vi "APS Controller.vi"() -> ()   [LabVIEW 2025]
panel:
  in  "Polarity":enum16{"Positive", "Negative"}(ring)
  out "Current Setpoint":i32
  in  "APS PORT":refnum<visa-resource-name>="COM3"
  out "?":string
  out "error out":errorcluster
  out "Connected?":bool
  in  "Set current":i32
  in  "Set Voltage":i32
  in  "Measure Temp":bool
  in  "Measure AUX2":bool
  in  "Measure AUX1":bool
  in  "Connect":bool
  in  "Stop Button":bool
  in  "Measure Voltage":bool
  in  "Measure Current":bool
  in  "Set INT Mode":bool
  in  "Set Current":bool
  in  "Set PC Mode":bool
  in  "Set Voltage":bool
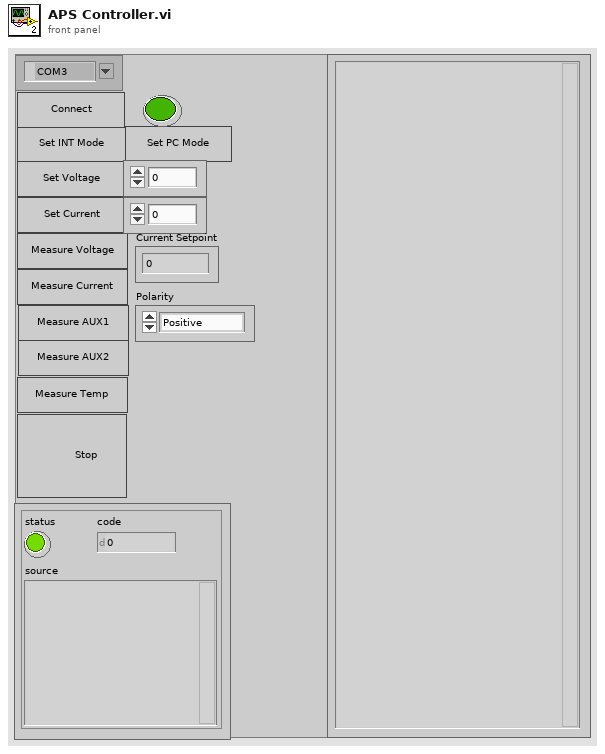
[diagram p1: front panel]
types:
  T1 = enum16{"1. Identify", "2. Control Mode", "3. Set PC Mode", "4. Set INT Mode", "5. Set Voltage", "6. Set Current", "7. Measure Voltage", "8. Measure Current", "9. Measure AUX1", "10. Measure AUX2", "11. Measure Temperature", "12. Switch Polarity"}
  T2 = cluster{"Task Type":enum16{"1. Identify", "2. Control Mode", "3. Set PC Mode", "4. Set INT Mode", "5. Set Voltage", "6. Set Current", "7. Measure Voltage", "8. Measure Current", "9. Measure AUX1", "10. Measure AUX2", "11. Measure Temperature", "12. Switch Polarity"}, "DBL Argument":i32, "BLN Argument":bool, "Task CMD":enum16{"*IDN?", "CONT MODE?", "CONT MODE PC", "CONT MODE INT", "SOUR VOLT ", "SOUR CURR ", "MEAS VOLT?", "MEAS CURR?", "MEAS AUX1?", "MEAS AUX2?", "MEAS TEMP?", "SOUR POLA"}, "CMD TYPE":enum16{"1. Timeout?", "2. New Current?", "3. User CMD"}, "Polarity":enum16{"POS ", "NEG "}}
  T3 = enum16{"*IDN?", "CONT MODE?", "CONT MODE PC", "CONT MODE INT", "SOUR VOLT ", "SOUR CURR ", "MEAS VOLT?", "MEAS CURR?", "MEAS AUX1?", "MEAS AUX2?", "MEAS TEMP?", "SOUR POLA"}
  T4 = enum16{"*IDN?", "CONT MODE?", "CONT MODE PC", "CONT MODE INT", "SOUR VOLT ", "SOUR CURR ", "MEAS VOLT?", "MEAS CURR?", "MEAS AUX1?", "MEAS AUX2?", "MEAS TEMP?"}
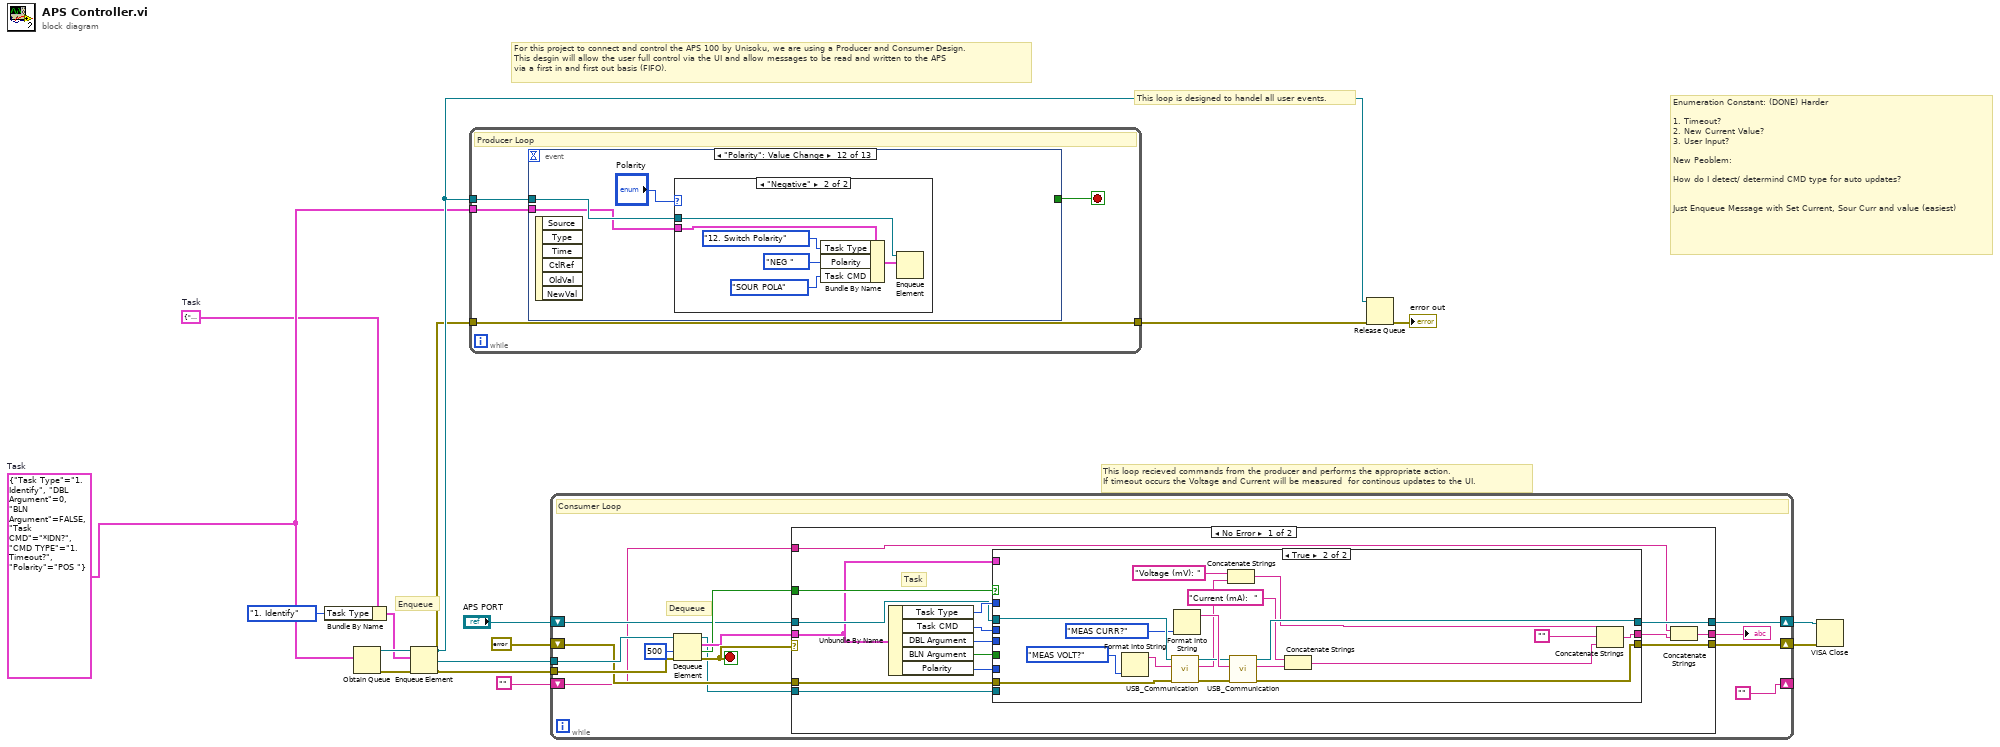
[diagram p0: block diagram]
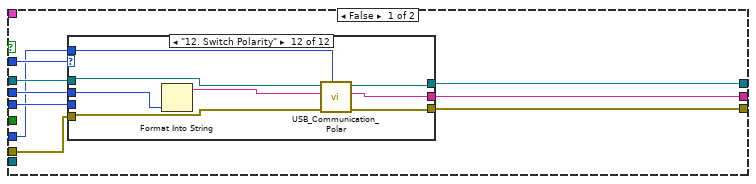
[diagram p2: hidden frame]
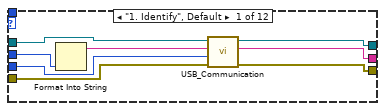
[diagram p3: hidden frame]
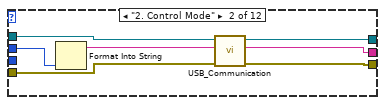
[diagram p4: hidden frame]
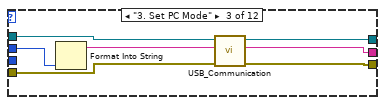
[diagram p5: hidden frame]
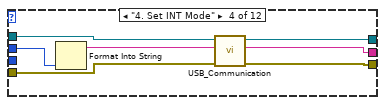
[diagram p6: hidden frame]
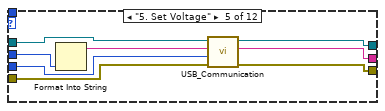
[diagram p7: hidden frame]
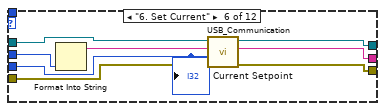
[diagram p8: hidden frame]
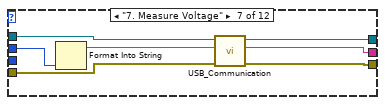
[diagram p9: hidden frame]
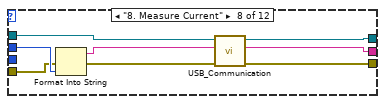
[diagram p10: hidden frame]
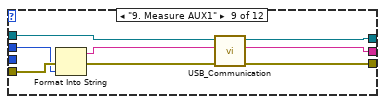
[diagram p11: hidden frame]
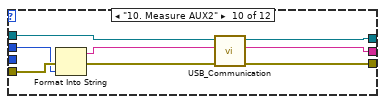
[diagram p12: hidden frame]
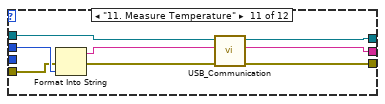
[diagram p13: hidden frame]
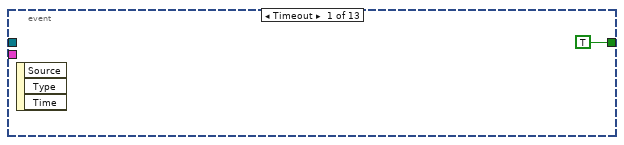
[diagram p15: hidden frame]
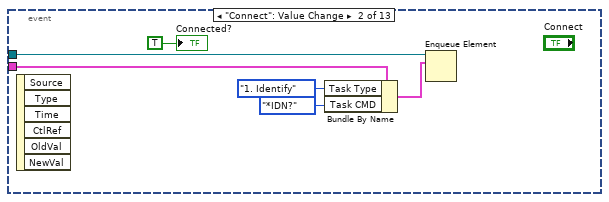
[diagram p16: hidden frame]
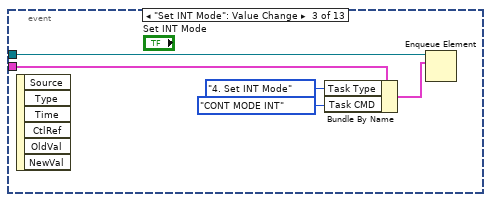
[diagram p17: hidden frame]
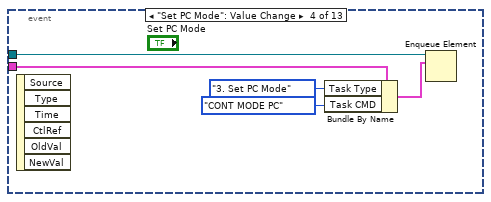
[diagram p18: hidden frame]
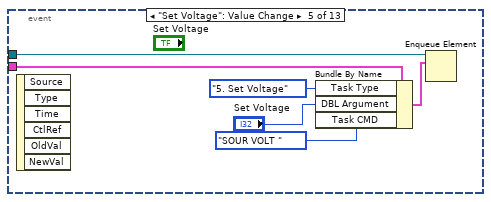
[diagram p19: hidden frame]
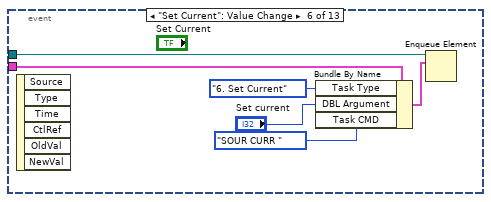
[diagram p20: hidden frame]
diagram:
  w3 = T2 {"Task Type"=enum."1. Identify", "DBL Argument"=0, "BLN Argument"=FALSE, "Task CMD"=enum."*IDN?", "CMD TYPE"=enum."1. Timeout?", "Polarity"=enum."POS "}  # Task
  w4 = T2 {"Task Type"=enum."1. Identify", "DBL Argument"=0, "BLN Argument"=FALSE, "Task CMD"=enum."*IDN?", "CMD TYPE"=enum."1. Timeout?", "Polarity"=enum."POS "}  # Task
  # "Enqueue"
  # "Enumeration Constant: (DONE) Harder\n\n1. Timeout?\n2. New Current Value?\n3. User Input? \n\nNew Peoblem:\n\nHow do I detect/ determind CMD type for auto updates?\n\n\nJust Enqueue Message with Set Current, Sour Curr and value (easiest)"
  # "This loop is designed to handel all user events."
  # "This loop recieved commands from the producer and performs the appropriate action.\nIf timeout occurs the Voltage and Current will be measured  for continous updates to the UI."
  # "For this project to connect and control the APS 100 by Unisoku, we are using a Producer and Consumer Design. \nThis desgin will allow the user full control via the UI and allow messages to be read and written to the APS\nvia a first in and first out basis (FIFO)."
  n1 = Bundle By Name(cluster=w3, "Task Type"=T1."1. Identify") -> (w1:T2)
  n2 = Obtain Queue(element data type=w4) -> (queue out=w5:refnum<queue>, error out=w15:errorcluster)  [unwired: 4 in, 1 out]
  n3 = Enqueue Element(queue=w5, element=w1, error in (no error)=w15) -> (queue out=w14:refnum<queue>, error out=w13:errorcluster)  [unwired: 1 in, 1 out]
  n4 = while {
    tunnel: w14 -> [w19]
    tunnel: w13 -> [w16]
    tunnel: w4 -> [w17]
    tunnel: [w16] -> w10
    stop <- w18 stop-if-true
    # "Producer Loop"
    n5 = event shown="[11] \"Polarity\": Value Change" {
      selector: _ -> [_ _ _ _ _ _ _ _ _ _ _ _ _]
      dyn-events: _ -> [_ _ _ _ _ _ _ _ _ _ _ _ _]
      timeout: _ -> [_ _ _ _ _ _ _ _ _ _ _ _ _]
      tunnel: w19 -> [_ w26 w29 w35 w39 w46 w51 w56 w61 w66 w71 w75 _]
      tunnel: [TRUE _ _ _ _ _ _ _ _ _ _ _ TRUE] -> w18
      tunnel: w17 -> [_ w25 w30 w34 w41 w47 w52 w57 w62 w67 w72 w74 _]
      event Timeout {
        n6 = event-data() -> ()  [unwired: 1 in, 3 out]
      }
      event "Connect": Value Change {
        n7 = event-data() -> ()  [unwired: 1 in, 6 out]
        n8 = Bundle By Name(cluster=w25, "Task Type"=T1."1. Identify", "Task CMD"=T3."*IDN?") -> (w24:T2)
        n9 = Enqueue Element(queue=w26, element=w24) -> ()  [unwired: 2 in, 3 out]
        "Connected?" <- TRUE
      }
      event "Set INT Mode": Value Change {
        n10 = event-data() -> ()  [unwired: 1 in, 6 out]
        n11 = Bundle By Name(cluster=w30, "Task Type"=T1."4. Set INT Mode", "Task CMD"=T3."CONT MODE INT") -> (w31:T2)
        n12 = Enqueue Element(queue=w29, element=w31) -> ()  [unwired: 2 in, 3 out]
      }
      event "Set PC Mode": Value Change {
        n13 = event-data() -> ()  [unwired: 1 in, 6 out]
        n14 = Bundle By Name(cluster=w34, "Task Type"=T1."3. Set PC Mode", "Task CMD"=T3."CONT MODE PC") -> (w36:T2)
        n15 = Enqueue Element(queue=w35, element=w36) -> ()  [unwired: 2 in, 3 out]
      }
      event "Set Voltage": Value Change {
        n16 = event-data() -> ()  [unwired: 1 in, 6 out]
        n17 = Bundle By Name(cluster=w41, "Task Type"=T1."5. Set Voltage", "DBL Argument"="Set Voltage", "Task CMD"=T3."SOUR VOLT ") -> (w42:T2)
        n18 = Enqueue Element(queue=w39, element=w42) -> ()  [unwired: 2 in, 3 out]
      }
      event "Set Current": Value Change {
        n19 = event-data() -> ()  [unwired: 1 in, 6 out]
        n20 = Bundle By Name(cluster=w47, "Task Type"=T1."6. Set Current", "DBL Argument"="Set current", "Task CMD"=T3."SOUR CURR ") -> (w48:T2)
        n21 = Enqueue Element(queue=w46, element=w48) -> ()  [unwired: 2 in, 3 out]
      }
      event "Measure Voltage": Value Change {
        n22 = event-data() -> ()  [unwired: 1 in, 6 out]
        n23 = Bundle By Name(cluster=w52, "Task Type"=T1."7. Measure Voltage", "Task CMD"=T3."MEAS VOLT?") -> (w53:T2)
        n24 = Enqueue Element(queue=w51, element=w53) -> ()  [unwired: 2 in, 3 out]
      }
      event "Measure Current": Value Change {
        n25 = event-data() -> ()  [unwired: 1 in, 6 out]
        n26 = Bundle By Name(cluster=w57, "Task Type"=T1."8. Measure Current", "Task CMD"=T3."MEAS CURR?") -> (w58:T2)
        n27 = Enqueue Element(queue=w56, element=w58) -> ()  [unwired: 2 in, 3 out]
      }
      event "Measure AUX1": Value Change {
        n28 = event-data() -> ()  [unwired: 1 in, 2 out]
        n29 = Bundle By Name(cluster=w62, "Task Type"=T1."9. Measure AUX1", "Task CMD"=T3."MEAS AUX1?") -> (w63:T2)
        n30 = Enqueue Element(queue=w61, element=w63) -> ()  [unwired: 2 in, 3 out]
      }
      event "Measure AUX2": Value Change {
        n31 = event-data() -> ()  [unwired: 1 in, 6 out]
        n32 = Bundle By Name(cluster=w67, "Task Type"=T1."10. Measure AUX2", "Task CMD"=T3."MEAS AUX2?") -> (w68:T2)
        n33 = Enqueue Element(queue=w66, element=w68) -> ()  [unwired: 2 in, 3 out]
      }
      event "Measure Temp": Value Change {
        n34 = event-data() -> ()  [unwired: 1 in, 6 out]
        n35 = Bundle By Name(cluster=w72, "Task Type"=T1."11. Measure Temperature", "Task CMD"=T3."MEAS TEMP?") -> (w73:T2)
        n36 = Enqueue Element(queue=w71, element=w73) -> ()  [unwired: 2 in, 3 out]
      }
      event "Polarity": Value Change {
        n37 = event-data() -> ()  [unwired: 1 in, 6 out]
        n38 = case shown="\"Negative\"" "Polarity" {
          tunnel: w75 -> [w82 w85]
          tunnel: w74 -> [w81 w84]
          frame "Positive", Default {
            n39 = Bundle By Name(cluster=w81, "Task Type"=T1."12. Switch Polarity", "Polarity"=enum16{"POS ", "NEG "}."POS ", "Task CMD"=T3."SOUR POLA") -> (w80:T2)
            n40 = Enqueue Element(queue=w82, element=w80) -> ()  [unwired: 2 in, 3 out]
          }
          frame "Negative" {
            n41 = Bundle By Name(cluster=w84, "Task Type"=T1."12. Switch Polarity", "Polarity"=enum16{"POS ", "NEG "}."NEG ", "Task CMD"=T3."SOUR POLA") -> (w88:T2)
            n42 = Enqueue Element(queue=w85, element=w88) -> ()  [unwired: 2 in, 3 out]
          }
        }
      }
      event "Stop Button": Value Change {
        n43 = event-data() -> ()  [unwired: 1 in, 6 out]
      }
    }
  }
  n44 = while {
    tunnel: w14 -> [w103]
    tunnel: w13 -> [w102]
    shift-right: [w96] -> w8
    shift-left: "APS PORT" -> [w98]
    shift-right: [w95] -> w7
    shift-left: errorcluster {"status"=FALSE, "code"=0, "source"=""} ("error in") -> [w97]
    shift-right: [""] -> _
    shift-left: "" -> [w94]
    stop <- w101 stop-if-true
    # "Dequeue"
    # "Consumer Loop"
    n45 = Dequeue Element(queue=w103, timeout in ms (-1)=500, error in (no error)=w102) -> (queue out=w90:refnum<queue>, element=w100:T2, timed out?=w99:bool, error out=w101:errorcluster)
    n46 = case shown="No Error" w101 {
      tunnel: w100 -> [w105 _]
      tunnel: w99 -> [w114 _]
      tunnel: w98 -> [w113 w239]
      tunnel: w97 -> [w112 w240]
      tunnel: [w111 w240] -> w95
      tunnel: [w110 w239] -> w96
      tunnel: w94 -> [w109 w238]
      tunnel: [w107 w238] -> w93
      tunnel: w90 -> [w106 _]
      frame No Error {
        # "Task"
        n47 = Unbundle By Name(w105) -> ("Task Type"=w118:T1, "Task CMD"=w117:T3, "DBL Argument"=w116:i32, "BLN Argument"=w115:bool, "Polarity"=w104:enum16{"POS ", "NEG "})
        n48 = case shown="True" w114 {
          tunnel: w118 -> [w127 _]
          tunnel: w117 -> [w125 _]
          tunnel: w116 -> [w121 _]
          tunnel: w115 -> [_ _]
          tunnel: w113 -> [w126 w236]
          tunnel: [w124 w229] -> w108
          tunnel: w112 -> [w123 w237]
          tunnel: [w120 w220] -> w111
          tunnel: [w122 w230] -> w110
          tunnel: w106 -> [_ _]
          tunnel: w105 -> [_ _]
          tunnel: w104 -> [w119 _]
          frame False {
            n49 = case shown="\"12. Switch Polarity\"" w127 {
              tunnel: w126 -> [w135 w141 w149 w155 w163 w172 w177 w184 w195 w201 w210 w218]
              tunnel: w125 -> [w134 w140 w148 w150 w161 w169 w179 w187 w191 w196 w211 w213]
              tunnel: [w132 w138 w143 w151 w159 w167 w173 w180 w189 w197 w206 w215] -> w124
              tunnel: w123 -> [w129 w142 w146 w154 w162 w171 w176 w183 w192 w200 w209 w217]
              tunnel: [w130 w137 w145 w152 w158 w166 w174 w181 w190 w198 w205 w216] -> w122
              tunnel: w121 -> [w128 _ _ _ w160 w168 _ _ _ _ _ _]
              tunnel: [w131 w136 w144 w153 w157 w165 w175 w182 w188 w199 w204 w214] -> w120
              tunnel: w119 -> [_ _ _ _ _ _ _ _ _ _ _ w212]
              frame "1. Identify", Default {
                n50 = Format Into String(w134) -> (resulting string=w133:string)  [unwired: 3 in, 1 out]
                n51 = call "USB_Communication.vi"("error in (no error)"=w129, "number"=w128, "string"=w133, "APS PORT"=w135) -> ("error out"=w131:errorcluster, "read buffer"=w132:string, "APS PORT Out"=w130:refnum<visa-resource-name>)  [unwired: 5 in]
              }
              frame "2. Control Mode" {
                n52 = Format Into String(w140) -> (resulting string=w139:string)  [unwired: 3 in, 1 out]
                n53 = call "USB_Communication.vi"("error in (no error)"=w142, "string"=w139, "APS PORT"=w141) -> ("error out"=w136:errorcluster, "read buffer"=w138:string, "APS PORT Out"=w137:refnum<visa-resource-name>)  [unwired: 6 in]
              }
              frame "3. Set PC Mode" {
                n54 = Format Into String(w148) -> (resulting string=w147:string)  [unwired: 3 in, 1 out]
                n55 = call "USB_Communication.vi"("error in (no error)"=w146, "string"=w147, "APS PORT"=w149) -> ("error out"=w144:errorcluster, "read buffer"=w143:string, "APS PORT Out"=w145:refnum<visa-resource-name>)  [unwired: 6 in]
              }
              frame "4. Set INT Mode" {
                n56 = Format Into String(w150) -> (resulting string=w156:string)  [unwired: 3 in, 1 out]
                n57 = call "USB_Communication.vi"("error in (no error)"=w154, "string"=w156, "APS PORT"=w155) -> ("error out"=w153:errorcluster, "read buffer"=w151:string, "APS PORT Out"=w152:refnum<visa-resource-name>)  [unwired: 6 in]
              }
              frame "5. Set Voltage" {
                n58 = Format Into String(w161) -> (resulting string=w164:string)  [unwired: 3 in, 1 out]
                n59 = call "USB_Communication.vi"("error in (no error)"=w162, "number"=w160, "string"=w164, "APS PORT"=w163) -> ("error out"=w157:errorcluster, "read buffer"=w159:string, "APS PORT Out"=w158:refnum<visa-resource-name>)  [unwired: 5 in]
              }
              frame "6. Set Current" {
                n60 = Format Into String(w169) -> (resulting string=w170:string)  [unwired: 3 in, 1 out]
                n61 = call "USB_Communication.vi"("error in (no error)"=w171, "number"=w168, "string"=w170, "APS PORT"=w172) -> ("error out"=w165:errorcluster, "read buffer"=w167:string, "APS PORT Out"=w166:refnum<visa-resource-name>)  [unwired: 5 in]
                "Current Setpoint" <- w168
              }
              frame "7. Measure Voltage" {
                n62 = Format Into String(w179) -> (resulting string=w178:string)  [unwired: 3 in, 1 out]
                n63 = call "USB_Communication.vi"("error in (no error)"=w176, "string"=w178, "APS PORT"=w177) -> ("error out"=w175:errorcluster, "read buffer"=w173:string, "APS PORT Out"=w174:refnum<visa-resource-name>)  [unwired: 6 in]
              }
              frame "8. Measure Current" {
                n64 = Format Into String(error in=w183, w187) -> (resulting string=w185:string, error out=w186:errorcluster)  [unwired: 2 in]
                n65 = call "USB_Communication.vi"("error in (no error)"=w186, "string"=w185, "APS PORT"=w184) -> ("error out"=w182:errorcluster, "read buffer"=w180:string, "APS PORT Out"=w181:refnum<visa-resource-name>)  [unwired: 6 in]
              }
              frame "9. Measure AUX1" {
                n66 = Format Into String(error in=w192, w191) -> (resulting string=w194:string, error out=w193:errorcluster)  [unwired: 2 in]
                n67 = call "USB_Communication.vi"("error in (no error)"=w193, "string"=w194, "APS PORT"=w195) -> ("error out"=w188:errorcluster, "read buffer"=w189:string, "APS PORT Out"=w190:refnum<visa-resource-name>)  [unwired: 6 in]
              }
              frame "10. Measure AUX2" {
                n68 = Format Into String(error in=w200, w196) -> (resulting string=w203:string, error out=w202:errorcluster)  [unwired: 2 in]
                n69 = call "USB_Communication.vi"("error in (no error)"=w202, "string"=w203, "APS PORT"=w201) -> ("error out"=w199:errorcluster, "read buffer"=w197:string, "APS PORT Out"=w198:refnum<visa-resource-name>)  [unwired: 6 in]
              }
              frame "11. Measure Temperature" {
                n70 = Format Into String(error in=w209, w211) -> (resulting string=w207:string, error out=w208:errorcluster)  [unwired: 2 in]
                n71 = call "USB_Communication.vi"("error in (no error)"=w208, "string"=w207, "APS PORT"=w210) -> ("error out"=w204:errorcluster, "read buffer"=w206:string, "APS PORT Out"=w205:refnum<visa-resource-name>)  [unwired: 6 in]
              }
              frame "12. Switch Polarity" {
                n72 = Format Into String(w213) -> (resulting string=w219:string)  [unwired: 3 in, 1 out]
                n73 = call "USB_Communication_Polar.vi"("Polarity"=w212, "error in (no error)"=w217, "string"=w219, "APS PORT"=w218) -> ("error out"=w214:errorcluster, "read buffer"=w215:string, "APS PORT Out"=w216:refnum<visa-resource-name>)  [unwired: 5 in]
              }
            }
          }
          frame True {
            n74 = Format Into String(T4."MEAS VOLT?" ("Task CMD")) -> (resulting string=w235:string)  [unwired: 3 in, 1 out]
            n75 = call "USB_Communication.vi"("error in (no error)"=w237, "string"=w235, "APS PORT"=w236) -> ("error out"=w227:errorcluster, "read buffer"=w225:string, "APS PORT Out"=w231:refnum<visa-resource-name>)  [unwired: 6 in]
            n76 = Format Into String(T4."MEAS CURR?" ("Task CMD")) -> (resulting string=w232:string)  [unwired: 3 in, 1 out]
            n77 = Concatenate Strings("Voltage (mV): " ("string"), w225) -> (w224:string)
            n78 = call "USB_Communication.vi"("error in (no error)"=w227, "string"=w232, "APS PORT"=w231) -> ("error out"=w220:errorcluster, "read buffer"=w223:string, "APS PORT Out"=w230:refnum<visa-resource-name>)  [unwired: 6 in]
            n79 = Concatenate Strings("Current (mA):  " ("string"), w223) -> (w221:string)
            n80 = Concatenate Strings(w224, "", w221) -> (w229:string)
          }
        }
        n81 = Concatenate Strings(w109, w108) -> (w107:string)
      }
      frame Error {
      }
    }
    "?" <- w93
  }
  n82 = Release Queue(queue=w14, error in (no error)=w10) -> (error out=→"error out":errorcluster)  [unwired: 1 in, 2 out]
  n83 = VISA Close(VISA resource name=w8, error in (no error)=w7) -> ()  [unwired: 1 out]
